vi "Discover Plugin Types.vi"(6 "timeout (ms)":i32=5000, 8 "error in (no error)":errorcluster, 10 "reload":bool, 11 "CIF_UI in":refnum<class "CIF_UI.lvclass">) -> (0 "error out":errorcluster, 3 "CIF_UI out":refnum<class "CIF_UI.lvclass">)   [LabVIEW 2021, in "CIF_UI.lvclass"]
uses:
  CIF_UI.lvclass
  CIF_UI.lvclass/CIF_UI.ctl
  CIFPluginManager/CIFPluginManager/gRPC/CIF_Manager_Client_Wrapper/CIFManagerClientWrapper.lvlib
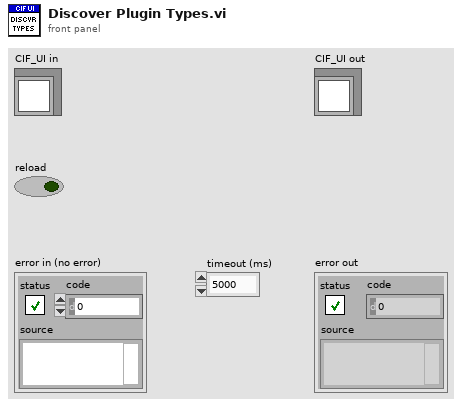
[diagram p1: front panel]
types:
  T1 = typedef "grpc-lvsupport-release.lvlib/grpcId.ctl" = u64
  T2 = typedef "CIF_Manager_client.lvlib/cif_manager_PluginType.ctl" = cluster{"plugin_type":string, "plugin_version":T3, "plugin_metadata":T4}
  T3 = typedef "CIF_Manager_client.lvlib/cif_common_ShortVersion.ctl" = cluster{"major":u32, "minor":u32, "fix":u32}
  T4 = typedef "CIF_Manager_client.lvlib/cif_manager_PluginMetadata.ctl" = cluster{"description":string, "history":string, "author":string}
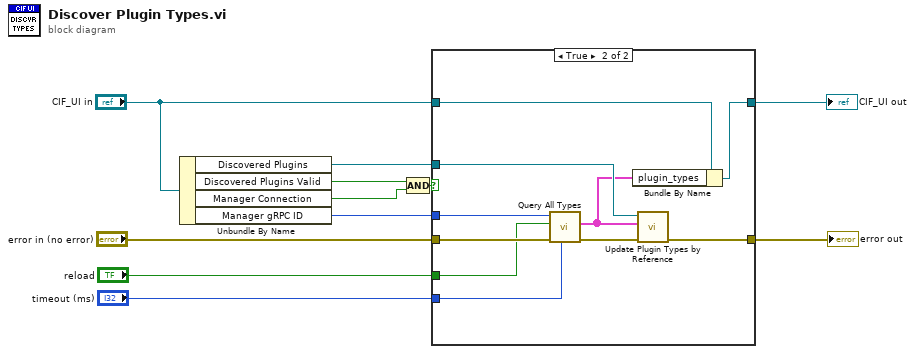
[diagram p0: block diagram]
diagram:
  n1 = Unbundle By Name("CIF_UI in") -> ("Discovered Plugins"=w7:refnum<vi>, "Discovered Plugins Valid"=w8:bool, "Manager Connection"=w5:bool, "Manager gRPC ID"=w6:T1)
  n2 = Compound Arithmetic op=AND(w8, w5) -> (w10:bool)
  n3 = case shown="True" w10 {
    tunnel: "error in (no error)" -> [w13 w23]
    tunnel: [w13 w22] -> w11
    tunnel: w6 -> [_ w20]
    tunnel: w7 -> [_ w19]
    tunnel: "CIF_UI in" -> [w12 w18]
    tunnel: [w12 w16] -> w3
    tunnel: "reload" -> [_ w15]
    tunnel: "timeout (ms)" -> [_ w14]
    frame False {
    }
    frame True {
      n4 = call "Query All Types.vi"("timeout (ms)"=w14, "error in"=w23, "reload"=w15, "gRPC ID in"=w20) -> ("error out"=w21:errorcluster, "plugin_types"=w17:T2[])  [unwired: 5 in, 1 out]
      n5 = Bundle By Name(cluster=w18, "plugin_types"=w17) -> (w16:refnum<class "CIF_UI.lvclass">)
      n6 = call "Update Plugin Types by Reference.vi"("error in (no error)"=w21, "plugin_types"=w17, "Plugin Types ref in"=w19) -> ("error out"=w22:errorcluster)  [unwired: 7 in, 1 out]
    }
  }
  "error out" <- w11
  "CIF_UI out" <- w3
